vi "Evaluate Status.vi"(8 "error in (no error)":errorcluster, 11 "Project Builder in":refnum<class "Project Builder.lvclass">) -> (0 "error out":errorcluster, 1 "Passed?":bool, 3 "Project Builder out":refnum<class "Project Builder.lvclass">)   [LabVIEW 2019, in "ProjectBuilder.lvlib" / "Project Builder.lvclass"]
doc: "Evaluate results and store the result in Status.txt in the report folder (if the path is not empty)."
uses:
  Project Builder.lvclass
  <vilib>/Utility/file.llb/Write Delimited Spreadsheet (string).vi
  Data/Report Data/Report Data.lvclass
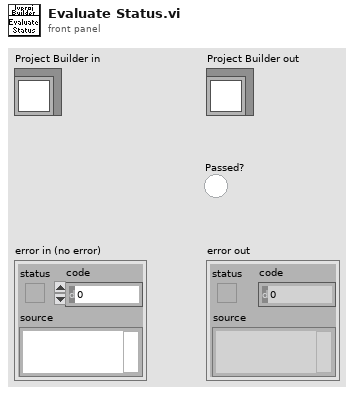
[diagram p1: front panel]
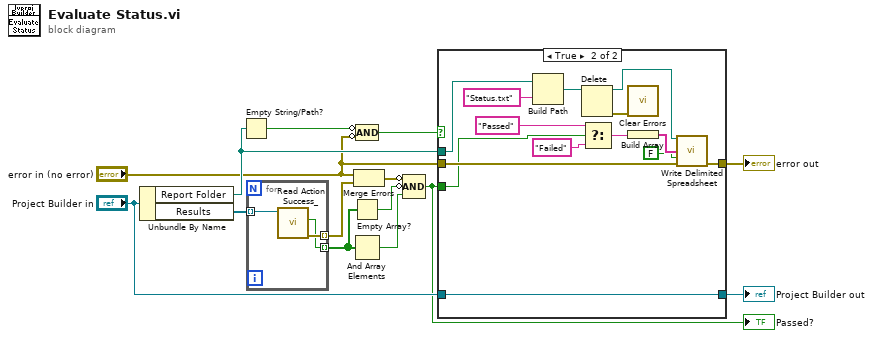
[diagram p0: block diagram]
diagram:
  n1 = Unbundle By Name("Project Builder in") -> ("Report Folder"=w9:path, "Results"=w8:refnum<class "Report Data.lvclass">[])
  n2 = Empty String/Path?(string/path=w9) -> (empty?=w11:bool)
  n3 = for {
    tunnel: w8 -> [w17] mode=indexing
    tunnel: [w16] -> w7 mode=indexing
    tunnel: [w15] -> w5 mode=indexing
    n4 = call "Read Action Success_.vi"("Report Data in"=w17) -> ("error out"=w16:errorcluster, "Action Success?"=w15:bool)  [unwired: 8 in, 1 out]
  }
  n5 = Empty Array?(array=w5) -> (empty?=w4:bool)
  n6 = And Array Elements(Boolean array=w5) -> (logical AND=w3:bool)
  n7 = Merge Errors("error in (no error)", w7) -> (w1:errorcluster)
  n8 = Compound Arithmetic op=AND(invert w11, invert "error in (no error)") -> (w10:bool)
  n9 = Compound Arithmetic op=AND(invert w1, invert w4, w3) -> (w2:bool)
  "Passed?" <- w2
  n10 = case shown="True" w10 {
    tunnel: [w19 w25] -> w14
    tunnel: [w18 w33] -> w12
    tunnel: "Project Builder in" -> [w18 w33]
    tunnel: "error in (no error)" -> [w19 w32]
    tunnel: w9 -> [_ w31]
    tunnel: w2 -> [_ w20]
    frame False {
    }
    frame True {
      n11 = Build Path(base path=w31, name or relative path="Status.txt") -> (appended path=w22:path)
      n12 = Delete(path (use dialog)=w22) -> (deleted path=w21:path, error out=w23:errorcluster)  [unwired: 4 in, 1 out]
      n13 = Select(t="Passed", s=w20, f="Failed") -> (s? t:f=w27:string)
      n14 = call <vilib>:"Clear Errors.vi"("error in (no error)"=w23) -> ()  [unwired: 5 in, 2 out]
      n15 = Build Array(w27) -> (w26:string[])
      n16 = call-poly <vilib>:"Write Delimited Spreadsheet.vi"("file path (dialog if empty)"=w21, "1D data"=w26, "append to file? (new file:F)"=FALSE, "error in (no error)"=w32) -> ("error out"=w25:errorcluster)  [unwired: 10 in, 1 out]
    }
  }
  "error out" <- w14
  "Project Builder out" <- w12
